vi "JKISM++ Duplicate Modules.vi"() -> ()   [LabVIEW 2014]
uses:
  user.lib/_NEVSTOP/JKI State Machine++/_Support/JKISMQ/_JKISMQFGV.vi
  user.lib/_NEVSTOP/JKI State Machine++/JKI State Machine++.lvlib
panel:
  out "Module Names":string[](array[string])
  in  "List Module":bool
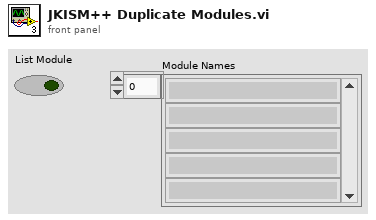
[diagram p1: front panel]
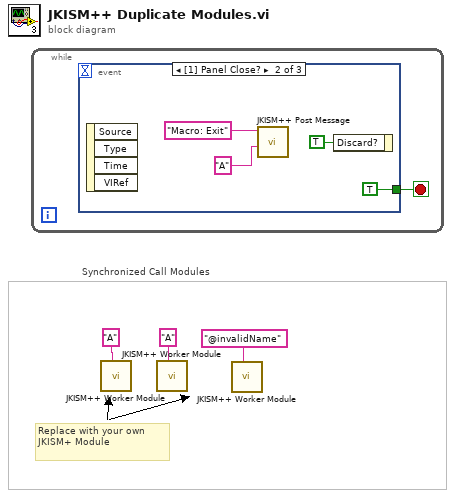
[diagram p0: block diagram]
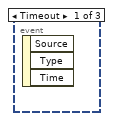
[diagram p2: hidden frame]
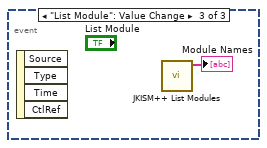
[diagram p3: hidden frame]
diagram:
  # "Replace with your own JKISM+ Module"
  # "Synchronized Call Modules"
  n1 = while {
    stop <- w4 stop-if-true
    n2 = event shown="[1] Panel Close?" {
      selector: _ -> [_ _ _]
      dyn-events: _ -> [_ _ _]
      timeout: _ -> [_ _ _]
      tunnel: [_ TRUE ("Discard?") _] -> w4
      event Timeout {
        n3 = event-data() -> ()  [unwired: 1 in, 3 out]
      }
      event Panel Close? {
        n4 = event-data() -> ()  [unwired: 1 in, 4 out]
        n5 = call "JKISM++ Post Message.vi"("Target Module"="A" ("Name"), "State"="Macro: Exit" ("Name")) -> ()  [unwired: 9 in, 1 out]
        n6 = event-data("Discard?"=TRUE) -> ()  [unwired: 1 in, 1 out]
      }
      event "List Module": Value Change {
        n7 = event-data() -> ()  [unwired: 1 in, 4 out]
        n8 = call "JKISM++ List Modules.vi"() -> ("Module Names"=→"Module Names":string[])  [unwired: 10 in, 1 out]
      }
    }
  }
  n9 = call "JKISM++ Worker Module.vi"("Name(\"\" to use uuid)"="A" ("Name")) -> ()  [unwired: 11 in]
  n10 = call "JKISM++ Worker Module.vi"("Name(\"\" to use uuid)"="A" ("Name")) -> ()  [unwired: 11 in]
  n11 = call "JKISM++ Worker Module.vi"("Name(\"\" to use uuid)"="@invalidName" ("Name")) -> ()  [unwired: 11 in]
